vi "Untitled 3.vi"() -> ()   [LabVIEW 2018]
panel:
  out "LS":dbl
  out "LI":dbl
  in  "vn":dbl format="%#_2p"
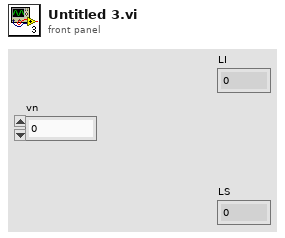
[diagram p1: front panel]
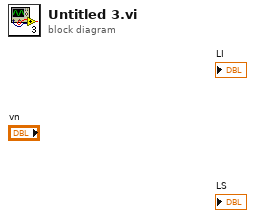
[diagram p0: block diagram]
diagram:
